vi "TPG361 status byte to msg (SubVI).vi"(8 "error in":errorcluster, 11 "In Error number":dbl) -> (0 "error out":errorcluster, 2 "Статус сообщение":string)   [LabVIEW 2014]
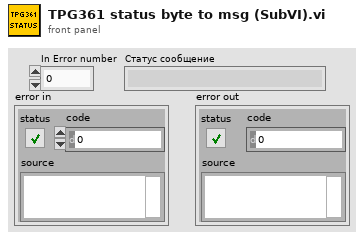
[diagram p1: front panel]
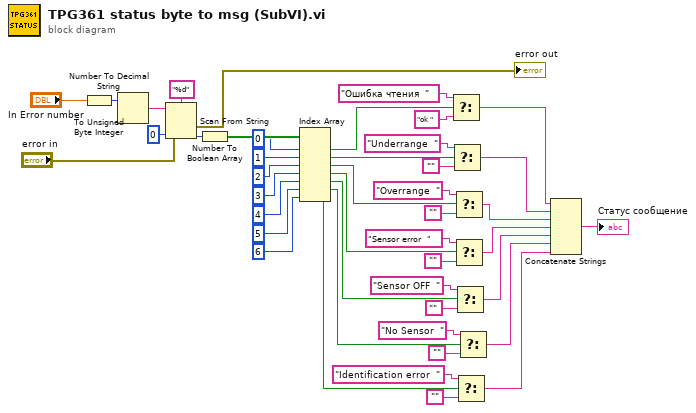
[diagram p0: block diagram]
diagram:
  n1 = To Unsigned Byte Integer(number="In Error number") -> (unsigned 8bit integer=w16:u8)
  n2 = Number To Decimal String(number=w16) -> (decimal integer string=w17:string)  [unwired: 1 in]
  n3 = Scan From String(format string="%d", input string=w17, error in="error in", default 1=u8 0 ("default value 1")) -> (error out=→"error out":errorcluster, output 1=w7:u8)  [unwired: 1 in, 2 out]
  n4 = Number To Boolean Array(number=w7) -> (Boolean array=w6:bool[])
  n5 = Index Array(array=w6, index #1=0 ("index"), index #2=1 ("index"), index #3=2 ("index"), index #4=3 ("index"), index #5=4 ("index"), index #6=5 ("index"), index #7=6 ("index")) -> (element #1=w14:bool, element #2=w19:bool, element #3=w23:bool, element #4=w26:bool, element #5=w29:bool, element #6=w32:bool, element #7=w35:bool)
  n6 = Select(t="Ошибка чтения  " ("format string"), s=w14, f="ok " ("format string")) -> (s? t:f=w37:string)
  n7 = Select(t="Underrange  " ("format string"), s=w19, f="") -> (s? t:f=w38:string)
  n8 = Select(t="Overrange  " ("format string"), s=w23, f="") -> (s? t:f=w39:string)
  n9 = Select(t="Sensor error  " ("format string"), s=w26, f="") -> (s? t:f=w40:string)
  n10 = Select(t="Sensor OFF  " ("format string"), s=w29, f="") -> (s? t:f=w41:string)
  n11 = Select(t="Identification error  " ("format string"), s=w35, f="") -> (s? t:f=w43:string)
  n12 = Select(t="No Sensor  " ("format string"), s=w32, f="") -> (s? t:f=w42:string)
  n13 = Concatenate Strings(w37, w38, w39, w40, w41, w42, w43) -> (→"Статус сообщение":string)
